vi "InitSpriteBuffer.vi"() -> ()   [LabVIEW 2019, in "Initializers.lvlib"]
uses:
  Initializers.lvlib
panel:
  out "new picture 3":picture
  out "new picture 2":picture
  in  "path to PNG file 3":path=path "C:/Users/FreshBob/Dropbox/VIs/myRIO_GameConsole/Data/Sprite3.png"
  in  "path to PNG file 2":path=path "C:/Users/FreshBob/Dropbox/VIs/myRIO_GameConsole/Data/Sprite2.png"
  out "new picture":picture
  in  "path to PNG file":path=path "C:/Users/FreshBob/Dropbox/VIs/myRIO_GameConsole/Data/Sprite1.png"
  out "Init Data Out":fxp<+,3,3>[](array[numeric])
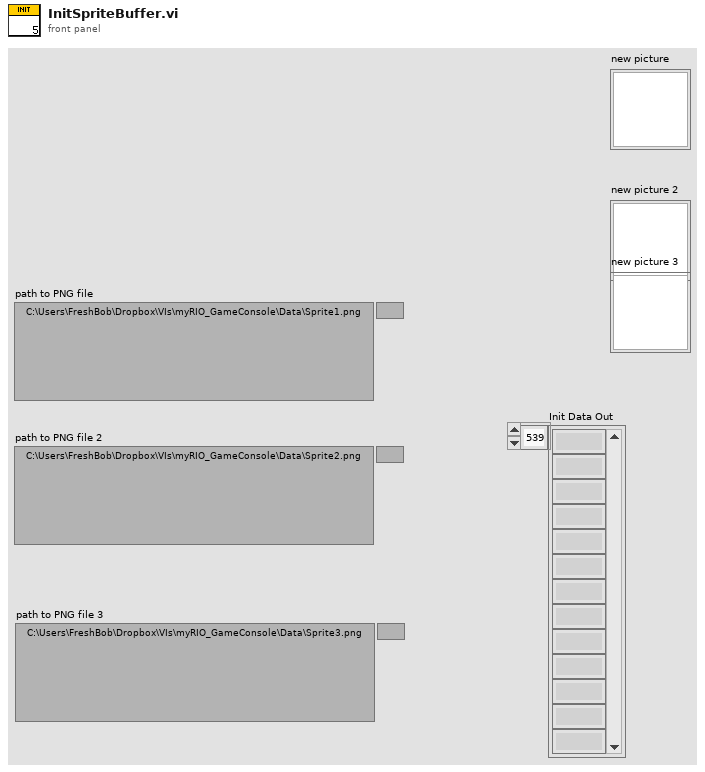
[diagram p1: front panel]
types:
  T1 = typedef "imagedata.ctl" = cluster{"image type":i32, "image depth":i32, "image":u8[], "mask":u8[], "colors":u32[], "Rectangle":cluster{"left":i16, "top":i16, "right":i16, "bottom":i16}}
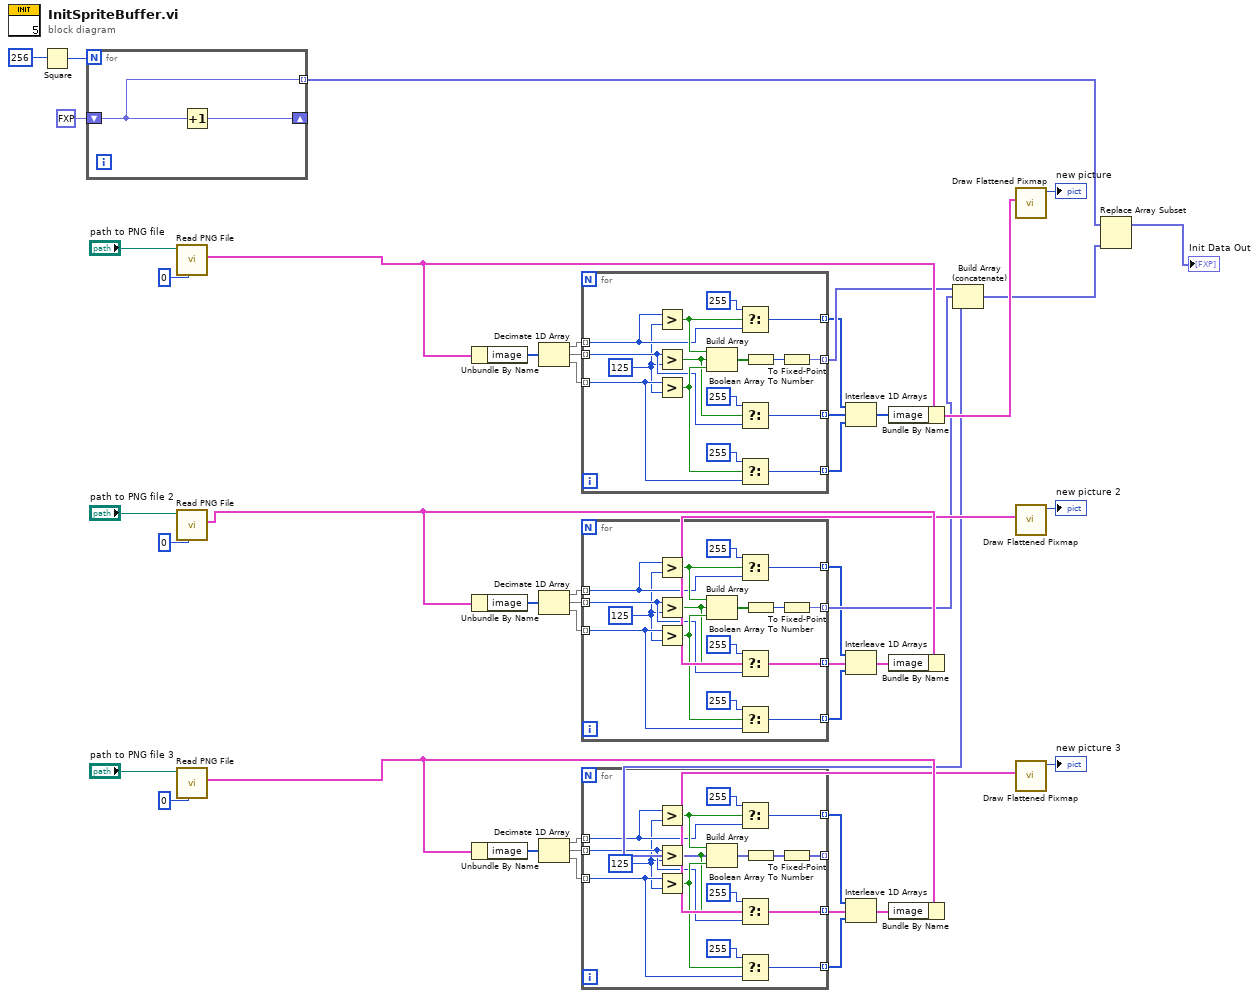
[diagram p0: block diagram]
diagram:
  n1 = Square(x=256) -> (x^2=w29:i32)
  n2 = for {
    N: w29 -> [_]
    shift-right: [w50] -> _
    shift-left: fxp<+,3,3> 0.0 -> [w49]
    tunnel: [w49] -> w27 mode=indexing
    n3 = Increment(x=w49) -> (x+1=w50:fxp<+,3,3>)
  }
  n4 = call <vilib>:"Read PNG File.vi"("Transparency Thresh"=u8 0, "path to PNG file"="path to PNG file") -> ("image data"=w46:T1)  [unwired: 7 in, 2 out]
  n5 = call <vilib>:"Read PNG File.vi"("Transparency Thresh"=u8 0, "path to PNG file"="path to PNG file 2") -> ("image data"=w39:T1)  [unwired: 7 in, 2 out]
  n6 = call <vilib>:"Read PNG File.vi"("Transparency Thresh"=u8 0, "path to PNG file"="path to PNG file 3") -> ("image data"=w38:T1)  [unwired: 7 in, 2 out]
  n7 = Unbundle By Name(w46) -> ("image"=w20:u8[])
  n8 = Unbundle By Name(w39) -> ("image"=w12:u8[])
  n9 = Unbundle By Name(w38) -> ("image"=w4:u8[])
  n10 = Decimate 1D Array(w20) -> (w19:u8[], w18:u8[], w17:u8[])
  n11 = Decimate 1D Array(w12) -> (w11:u8[], w10:u8[], w9:u8[])
  n12 = Decimate 1D Array(w4) -> (w3:u8[], w2:u8[], w1:u8[])
  n13 = for {
    tunnel: w19 -> [w55] mode=indexing
    tunnel: w18 -> [w59] mode=indexing
    tunnel: w17 -> [w58] mode=indexing
    tunnel: [w64] -> w33 mode=indexing
    tunnel: [w53] -> w22 mode=indexing
    tunnel: [w52] -> w23 mode=indexing
    tunnel: [w51] -> w24 mode=indexing
    w54 = u8 125 ("y")
    n14 = Greater?(x=w55, y=w54) -> (0:w63:bool)
    n15 = Greater?(x=w59, y=w54) -> (0:w61:bool)
    n16 = Greater?(x=w58, y=w54) -> (0:w62:bool)
    n17 = Build Array(w63, w61, w62) -> (w66:bool[])
    n18 = Select(t=u8 255, s=w63, f=w55) -> (s? t:f=w53:u8)
    n19 = Select(t=u8 255, s=w61, f=w59) -> (s? t:f=w52:u8)
    n20 = Select(t=u8 255, s=w62, f=w58) -> (s? t:f=w51:u8)
    n21 = Boolean Array To Number(Boolean array=w66) -> (number=w65:u32)
    n22 = To Fixed-Point(number=w65) -> (fixed-point=w64:fxp<+,3,3>)  [unwired: 1 in]
  }
  n23 = for {
    tunnel: w11 -> [w71] mode=indexing
    tunnel: w10 -> [w75] mode=indexing
    tunnel: w9 -> [w74] mode=indexing
    tunnel: [w80] -> w32 mode=indexing
    tunnel: [w69] -> w14 mode=indexing
    tunnel: [w68] -> w15 mode=indexing
    tunnel: [w67] -> w16 mode=indexing
    w70 = u8 125 ("y")
    n24 = Greater?(x=w71, y=w70) -> (0:w79:bool)
    n25 = Greater?(x=w75, y=w70) -> (0:w77:bool)
    n26 = Greater?(x=w74, y=w70) -> (0:w78:bool)
    n27 = Build Array(w79, w77, w78) -> (w82:bool[])
    n28 = Select(t=u8 255, s=w79, f=w71) -> (s? t:f=w69:u8)
    n29 = Select(t=u8 255, s=w77, f=w75) -> (s? t:f=w68:u8)
    n30 = Select(t=u8 255, s=w78, f=w74) -> (s? t:f=w67:u8)
    n31 = Boolean Array To Number(Boolean array=w82) -> (number=w81:u32)
    n32 = To Fixed-Point(number=w81) -> (fixed-point=w80:fxp<+,3,3>)  [unwired: 1 in]
  }
  n33 = for {
    tunnel: w3 -> [w87] mode=indexing
    tunnel: w2 -> [w91] mode=indexing
    tunnel: w1 -> [w90] mode=indexing
    tunnel: [w96] -> w31 mode=indexing
    tunnel: [w85] -> w6 mode=indexing
    tunnel: [w84] -> w7 mode=indexing
    tunnel: [w83] -> w8 mode=indexing
    w86 = u8 125 ("y")
    n34 = Greater?(x=w87, y=w86) -> (0:w95:bool)
    n35 = Greater?(x=w91, y=w86) -> (0:w93:bool)
    n36 = Greater?(x=w90, y=w86) -> (0:w94:bool)
    n37 = Build Array(w95, w93, w94) -> (w98:bool[])
    n38 = Select(t=u8 255, s=w95, f=w87) -> (s? t:f=w85:u8)
    n39 = Select(t=u8 255, s=w93, f=w91) -> (s? t:f=w84:u8)
    n40 = Select(t=u8 255, s=w94, f=w90) -> (s? t:f=w83:u8)
    n41 = Boolean Array To Number(Boolean array=w98) -> (number=w97:u32)
    n42 = To Fixed-Point(number=w97) -> (fixed-point=w96:fxp<+,3,3>)  [unwired: 1 in]
  }
  n43 = Interleave 1D Arrays(w22, w23, w24) -> (w21:u8[])
  n44 = Interleave 1D Arrays(w14, w15, w16) -> (w13:u8[])
  n45 = Interleave 1D Arrays(w6, w7, w8) -> (w5:u8[])
  n46 = Bundle By Name(cluster=w46, "image"=w21) -> (w45:T1)
  n47 = Bundle By Name(cluster=w39, "image"=w13) -> (w35:T1)
  n48 = Bundle By Name(cluster=w38, "image"=w5) -> (w34:T1)
  n49 = Build Array (concatenate)(w33, w32, w31) -> (w26:fxp<+,3,3>[])
  n50 = call <vilib>:"Draw Flattened Pixmap.vi"("image data"=w45) -> ("new picture"=→"new picture":picture)  [unwired: 8 in]
  n51 = call <vilib>:"Draw Flattened Pixmap.vi"("image data"=w35) -> ("new picture"=→"new picture 2":picture)  [unwired: 8 in]
  n52 = call <vilib>:"Draw Flattened Pixmap.vi"("image data"=w34) -> ("new picture"=→"new picture 3":picture)  [unwired: 8 in]
  n53 = Replace Array Subset(array=w27, new element=w26) -> (→"Init Data Out":fxp<+,3,3>[])  [unwired: 1 in]
